vi "tm3samp_01b_softwaretriggerbutton.vi"() -> ()   [LabVIEW 2023]
panel:
  in  "Quit":bool
  in  "About":bool
  in  "Snap":bool
  out "Image":u16[][](graph)
  out "Error Out":errorcluster
  # "This is a method to capture multiple frames without reallocating the buffer."
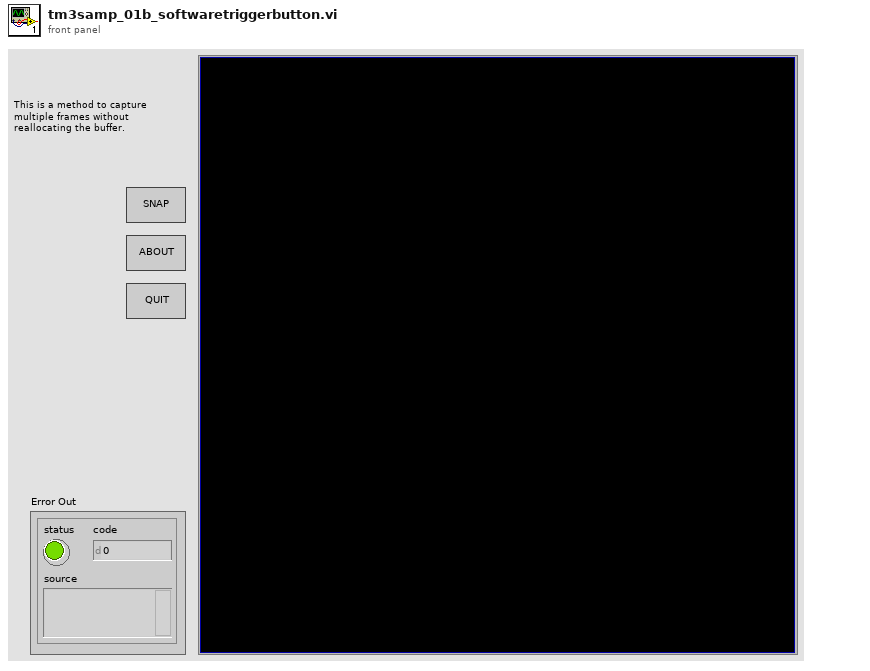
[diagram p1: front panel]
types:
  T1 = cluster{"Mode":u32, "Polarity":u32, "Times":u32, "Delay":dbl}
  T2 = cluster{"height":u32, "width":u32, "datatype":u32}
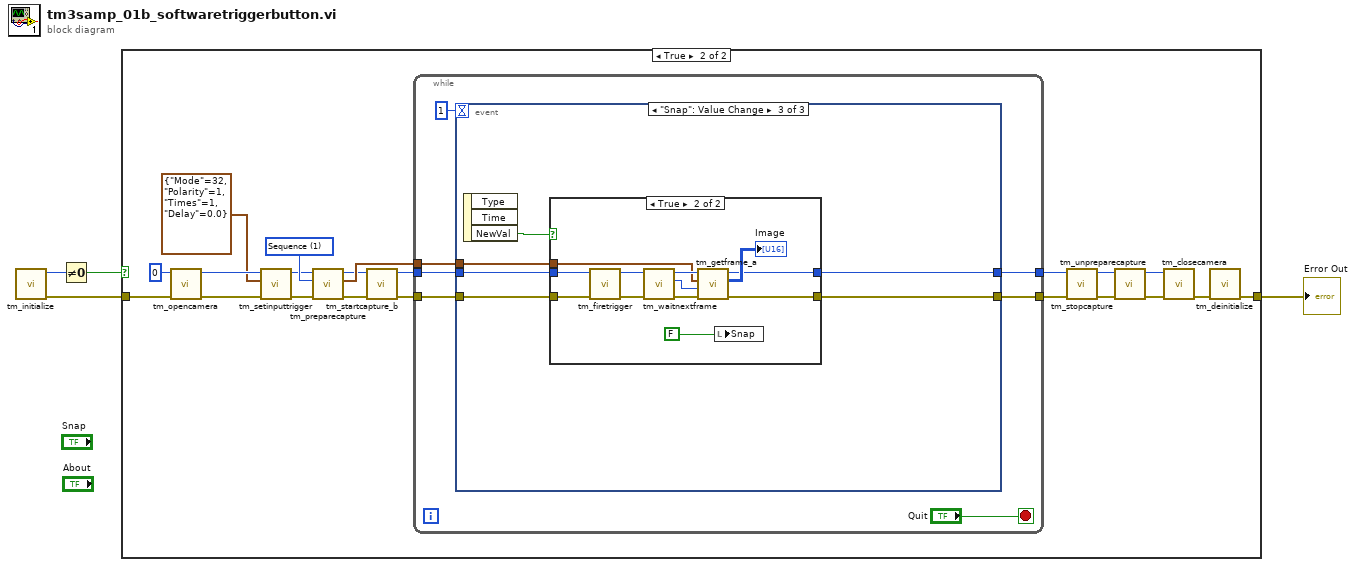
[diagram p0: block diagram]
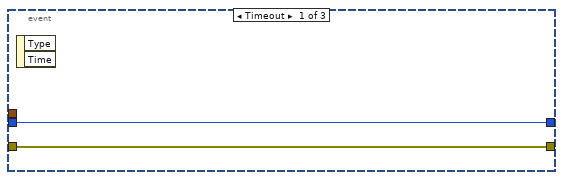
[diagram p3: hidden frame]
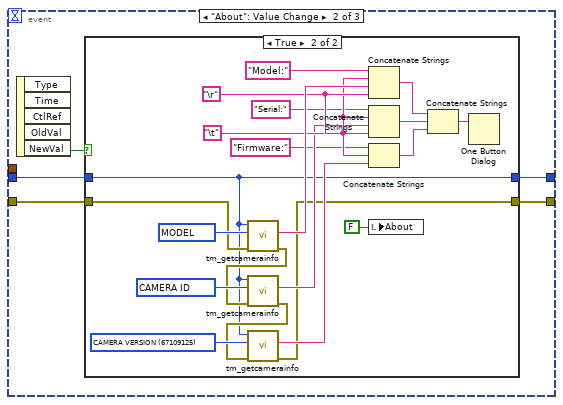
[diagram p4: hidden frame]
diagram:
  n1 = call "tm_initialize.vi"() -> ("error out"=w1:errorcluster, "Number Of Cameras"=w2:u32)  [unwired: 8 in, 2 out]
  n2 = Not Equal To 0?(x=w2) -> (x != 0?=w4:bool)
  n3 = case shown="True" w4 {
    tunnel: w1 -> [w5 w26]
    tunnel: [w5 w23] -> w3
    frame False {
    }
    frame True {
      w18 = 1 items=["Snap", "Sequence"] ("Capture mode")
      n4 = call "tm_opencamera.vi"("error in (no error)"=w26, "Camera Index"=u32 0) -> ("error out"=w9:errorcluster, "Handle out"=w10:u32)  [unwired: 7 in, 1 out]
      n5 = call "tm_setinputtrigger.vi"("error in (no error)"=w9, "Parameters"=T1 {"Mode"=32, "Polarity"=1, "Times"=1, "Delay"=0.0}, "Handle in"=w10) -> ("error out"=w7:errorcluster, "Handle out"=w8:u32)  [unwired: 7 in]
      n6 = call "tm_preparecapture.vi"("error in (no error)"=w7, "Capture mode"=w18, "Handle in"=w8) -> ("error out"=w14:errorcluster, "Buffer Info"=w17:T2, "Handle out"=w13:u32)  [unwired: 5 in, 1 out]
      n7 = call "tm_startcapture_b.vi"("error in (no error)"=w14, "Handle in"=w13) -> ("error out"=w11:errorcluster, "Handle out"=w12:u32)  [unwired: 8 in]
      n8 = while {
        tunnel: w12 -> [w31]
        tunnel: w17 -> [w32]
        tunnel: w11 -> [w33]
        tunnel: [w30] -> w16
        tunnel: [w29] -> w15
        stop <- "Quit" stop-if-true
        n9 = event shown="[2] \"Snap\": Value Change" {
          selector: _ -> [_ _ _]
          dyn-events: _ -> [_ _ _]
          timeout: 1 -> [_ _ _]
          tunnel: w33 -> [w34 w39 w69]
          tunnel: w31 -> [w35 w38 w67]
          tunnel: w32 -> [_ _ w66]
          tunnel: [w35 w36 w65] -> w30
          tunnel: [w34 w37 w64] -> w29
          event Timeout {
            n10 = event-data() -> ()  [unwired: 1 in, 2 out]
          }
          event "About": Value Change {
            n11 = event-data() -> ("NewVal"=w40:bool)  [unwired: 1 in, 4 out]
            n12 = case shown="True" w40 {
              tunnel: w39 -> [w41 w46]
              tunnel: w38 -> [w42 w44]
              tunnel: [w41 w45] -> w37
              tunnel: [w42 w44] -> w36
              frame False {
              }
              frame True {
                w55 = "\t"
                w56 = "\r"
                w63 = u32 67109122 items=["BUS"=67109121, "CAMERA ID"=67109122, "VENDOR"=67109123, "MODEL"=67109124, "CAMERA VERSION"=67109125, "DRIVER VERSION"=67109126, "MODULE VERSIOIN"=67109127, "DCAMAPI VERSION"=67109128] ("Info ID")
                w62 = u32 67109125 items=["BUS"=67109121, "CAMERA"=67109122, "VENDOR"=67109123, "MODEL"=67109124, "CAMERA VERSION"=67109125, "DRIVER VERSION"=67109126, "MODULE VERSIOIN"=67109127, "DCAMAPI VERSION"=67109128] ("Info ID")
                w59 = u32 67109124 items=["BUS"=67109121, "CAMERA"=67109122, "VENDOR"=67109123, "MODEL"=67109124, "CAMERA VERSION"=67109125, "DRIVER VERSION"=67109126, "MODULE VERSIOIN"=67109127, "DCAMAPI VERSION"=67109128] ("Info ID")
                n13 = call "tm_getcamerainfo.vi"("error in (no error)"=w46, "Info ID"=w59, "Handle in"=w44) -> ("error out"=w60:errorcluster, "String"=w57:string)  [unwired: 6 in, 1 out]
                n14 = call "tm_getcamerainfo.vi"("error in (no error)"=w60, "Info ID"=w63, "Handle in"=w44) -> ("error out"=w61:errorcluster, "String"=w53:string)  [unwired: 6 in, 1 out]
                n15 = call "tm_getcamerainfo.vi"("error in (no error)"=w61, "Info ID"=w62, "Handle in"=w44) -> ("error out"=w45:errorcluster, "String"=w54:string)  [unwired: 6 in, 1 out]
                n16 = Concatenate Strings("Model:", w55, w57, w56) -> (w50:string)
                n17 = Concatenate Strings("Serial:", w55, w53, w56) -> (w49:string)
                n18 = Concatenate Strings("Firmware:", w55, w54) -> (w48:string)
                n19 = local write "About"(FALSE ("About")) -> ()
                n20 = Concatenate Strings(w50, w49, w48) -> (w47:string)
                n21 = One Button Dialog(message=w47) -> ()  [unwired: 1 in, 1 out]
              }
            }
          }
          event "Snap": Value Change {
            n22 = event-data() -> ("NewVal"=w68:bool)  [unwired: 1 in, 2 out]
            n23 = case shown="True" w68 {
              tunnel: w69 -> [w70 w75]
              tunnel: w67 -> [w71 w74]
              tunnel: w66 -> [_ w79]
              tunnel: [w71 w78] -> w65
              tunnel: [w70 w77] -> w64
              frame False {
              }
              frame True {
                n24 = call "tm_firetrigger.vi"("error in (no error)"=w75, "Handle in"=w74) -> ("error out"=w72:errorcluster, "Handle out"=w73:u32)  [unwired: 8 in]
                n25 = call "tm_waitnextframe.vi"("error in (no error)"=w72, "Handle in"=w73) -> ("error out"=w82:errorcluster, "Frame Index"=w80:i32, "Handle out"=w81:u32)  [unwired: 6 in, 1 out]
                n26 = call "tm_getframe_a.vi"("error in (no error)"=w82, "Frame Index"=w80, "Buffer Info"=w79, "Handle in"=w81) -> ("error out"=w77:errorcluster, "Data 16"=→"Image":u16[][], "Handle out"=w78:u32)  [unwired: 3 in, 2 out]
                n27 = local write "Snap"(FALSE) -> ()
              }
            }
          }
        }
      }
      n28 = call "tm_stopcapture.vi"("error in (no error)"=w15, "Handle in"=w16) -> ("error out"=w19:errorcluster, "Handle out"=w20:u32)  [unwired: 8 in]
      n29 = call "tm_unpreparecapture.vi"("error in (no error)"=w19, "Handle in"=w20) -> ("error out"=w22:errorcluster, "Handle out"=w21:u32)  [unwired: 8 in]
      n30 = call "tm_closecamera.vi"("error in (no error)"=w22, "Handle in"=w21) -> ("error out"=w24:errorcluster)  [unwired: 9 in]
      n31 = call "tm_deinitialize.vi"("error in (no error)"=w24) -> ("error out"=w23:errorcluster)  [unwired: 10 in]
    }
  }
  "Error Out" <- w3
